vi "Read voltage.vi"(8 "error in (no error)":errorcluster, 11 "Component-A in":refnum<class "Component-A.lvclass">) -> (0 "error out":errorcluster, 2 "voltage":dbl, 3 "Component-A out":refnum<class "Component-A.lvclass">)   [LabVIEW 2018, in "Component-A.lvclass"]
uses:
  Component-A.lvclass
  Component-A.lvclass/Component-A.ctl
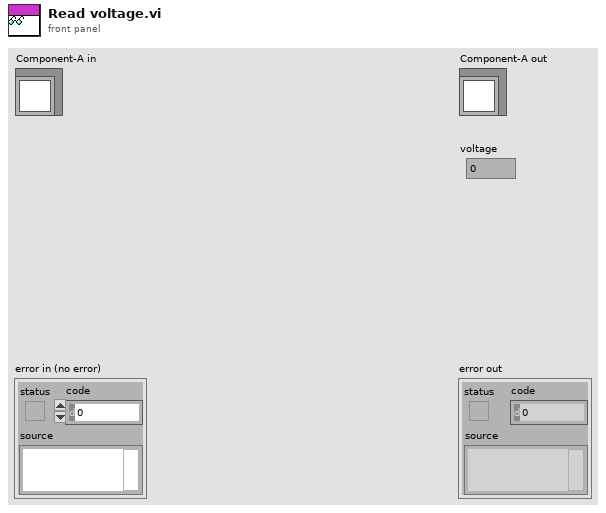
[diagram p1: front panel]
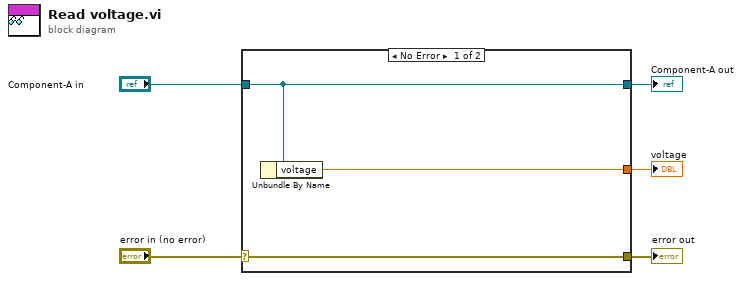
[diagram p0: block diagram]
diagram:
  n1 = case shown="No Error" "error in (no error)" {
    selector: "error in (no error)" -> [w8 w9]
    tunnel: [w8 w9] -> w4
    tunnel: [w7 w10] -> w2
    tunnel: "Component-A in" -> [w7 w10]
    tunnel: [w6 _] -> w1
    frame No Error {
      n2 = Unbundle By Name(w7) -> ("voltage"=w6:dbl)
    }
    frame Error {
    }
  }
  "error out" <- w4
  "Component-A out" <- w2
  "voltage" <- w1
